vi "ScanFSM_v2.vi"(0 "Scan XY Map References":T3, 4 "Scan XY Map Handles":T2, 10 "Params XY Map SubVI":T7, 12 "Scan XY Map Exp Params SubVI":T6) -> (13 "Handles Out":T1, 16 "Data":i32[][](array[numeric]))   [LabVIEW 2019]
uses:
  TypeDefs/AcqMode.ctl
  Light Field/lightfield-automation-labview/LightField Automation.lvclass
panel:
  out "size(s)":i32[](array[numeric])
  out "Numeric 2":i32
  out "Numeric":i32
  out "Number of points":dbl=121.0
  out "YMultiplier":dbl
  out "YOffset":dbl
  out "XMultiplier":dbl
  out "XOffset":dbl
  out "XYPos Indices Randomized":dbl[][](array[numeric])
  out "XYPos Indices":i32[][](array[numeric])
  out "Random index":i32[](array[numeric])=[4, 16, 17, 14, 92, 29, 8, 31, 42, 104, 84, 28, 85, 90, 13, 60, 120, 41, 111, 82, 69, 34, 7, 77, 47, 59, 65, 116, 24, 30, 113, 2, 63, 94, 106, 103, 71, 100, 22, 18, 32, 102, 19, 97, 44, 12, 0, 1, 109, 27, 88, 99, 51, 107, 76, 56, 81, 96, 72, 93, 74, 21, 5, 79, 9, 117, 38, 45, 25, 58, 105, 57, 40, 52, 23, 87, 89, 62, 26, 110, 37, 3, 101, 10, 54, 61, 83, 46, 86, 66, 68, 43, 108, 11, 67, 75, 6, 80, 49, 20, 112, 78, 115, 119, 95, 64, 73, 39, 15, 48, 55, 70, 50, 98, 91, 35, 53, 36, 118, 33, 114]
  out "X size":dbl=11.0
  out "Y size":dbl=11.0
  out "WL Calib":dbl[](array[numeric])
  out "LF Error Out":errorcluster
  out "LF Out":refnum<class "LightField Automation.lvclass">
  out "CCD 1D Spectrum XY Map":refnum<vi>
  out "CCD 1D Spectrum XY Map 2":cluster{dbl[], dbl[]}(graph)
  out "CCD ROI":T4(ring)
  out "Accumulations":dbl
  out "Acq Mode":T5=enum."Spectrum"
  out "KCube Shutter On?":bool
  out "A Time (ms)":dbl
  out "XY Intensity Map":refnum<vi>
  out "XY Intensity Map":dbl[][](graph)=[[3.904687043201515e-13, 6.684989195773002e-11, 3.649880430807626e-09, 6.355065252727497e-08, 3.5287820878809013e-07, 6.248749509463085e-07, 3.5287820878809013e-07, 6.355065252727497e-08, 3.649880430807626e-09, 6.684989195773002e-11, 3.904687043201515e-13], [6.684989195773002e-11, 1.1444983952148092e-08, 6.248749509463097e-07, 1.0880140221963334e-05, 6.041424029819161e-05, 0.0001069812317752422, 6.041424029819161e-05, 1.0880140221963334e-05, 6.248749509463097e-07, 1.1444983952148092e-08, 6.684989195773002e-11], [3.649880430807626e-09, 6.248749509463097e-07, 3.41170163237202e-05, 0.0005940355282204004, 0.003298505755939091, 0.005840977343195246, 0.003298505755939091, 0.0005940355282204004, 3.41170163237202e-05, 6.248749509463097e-07, 3.649880430807626e-09], [6.355065252727497e-08, 1.0880140221963334e-05, 0.0005940355282204004, 0.01034317319661825, 0.05743261926761737, 0.10170139230422684, 0.05743261926761737, 0.01034317319661825, 0.0005940355282204004, 1.0880140221963334e-05, 6.355065252727497e-08], [3.5287820878809013e-07, 6.041424029819161e-05, 0.003298505755939091, 0.05743261926761737, 0.31890655732397044, 0.5647181220077593, 0.31890655732397044, 0.05743261926761737, 0.003298505755939091, 6.041424029819161e-05, 3.5287820878809013e-07], [6.248749509463085e-07, 0.0001069812317752422, 0.005840977343195246, 0.10170139230422684, 0.5647181220077593, 1.0, 0.5647181220077593, 0.10170139230422684, 0.005840977343195246, 0.0001069812317752422, 6.248749509463085e-07], [3.5287820878809013e-07, 6.041424029819161e-05, 0.003298505755939091, 0.05743261926761737, 0.31890655732397044, 0.5647181220077593, 0.31890655732397044, 0.05743261926761737, 0.003298505755939091, 6.041424029819161e-05, 3.5287820878809013e-07], [6.355065252727497e-08, 1.0880140221963334e-05, 0.0005940355282204004, 0.01034317319661825, 0.05743261926761737, 0.10170139230422684, 0.05743261926761737, 0.01034317319661825, 0.0005940355282204004, 1.0880140221963334e-05, 6.355065252727497e-08], [3.649880430807626e-09, 6.248749509463097e-07, 3.41170163237202e-05, 0.0005940355282204004, 0.003298505755939091, 0.005840977343195246, 0.003298505755939091, 0.0005940355282204004, 3.41170163237202e-05, 6.248749509463097e-07, 3.649880430807626e-09], [6.684989195773002e-11, 1.1444983952148092e-08, 6.248749509463097e-07, 1.0880140221963334e-05, 6.041424029819161e-05, 0.0001069812317752422, 6.041424029819161e-05, 1.0880140221963334e-05, 6.248749509463097e-07, 1.1444983952148092e-08, 6.684989195773002e-11], [3.904687043201515e-13, 6.684989195773002e-11, 3.649880430807626e-09, 6.355065252727497e-08, 3.5287820878809013e-07, 6.248749509463085e-07, 3.5287820878809013e-07, 6.355065252727497e-08, 3.649880430807626e-09, 6.684989195773002e-11, 3.904687043201515e-13]]
  out "XY Map Elapsed (s)":refnum<vi>
  out "XY Map Expected (s)":refnum<vi>
  out "XY Map Expected (s)":dbl caption="Expected (s)"
  out "XY Map Elapsed (s)":dbl caption="Elapsed (s)"
  in  "DigNum Refnum":refnum<vi>
  out "Scan XY Map Progess Bar":refnum<vi>
  out "Stop XY Map":refnum<vi>
  in  "CCD 2D Image XY Map":refnum<vi>
  out "Scan Y Readout (V)":refnum<vi>
  out "Scan X Readout (V)":refnum<vi>
  out "XYPositions":dbl[][](array[numeric])=[[-0.09999999999999998, -0.3], [-0.09999999999999998, -0.19999999999999996], [-0.3, 0.4], [0.20000000000000007, -0.09999999999999998], [-0.5, -0.5], [0.0, 0.20000000000000007], [0.30000000000000004, 0.30000000000000004], [-0.3, -0.5], [-0.5, 0.10000000000000009], [0.0, 0.4], [0.20000000000000007, 0.10000000000000009], [0.30000000000000004, 0.0], [-0.09999999999999998, -0.4], [-0.4, -0.19999999999999996], [-0.5, -0.19999999999999996], [0.4, 0.4], [-0.5, -0.4], [-0.5, -0.3], [-0.19999999999999996, 0.10000000000000009], [-0.19999999999999996, 0.4], [0.4, -0.5], [0.0, 0.10000000000000009], [-0.19999999999999996, 0.0], [0.10000000000000009, 0.30000000000000004], [-0.3, 0.10000000000000009], [0.10000000000000009, -0.3], [0.20000000000000007, -0.4], [-0.09999999999999998, 0.0], [-0.4, -0.5], [-0.5, 0.0], [-0.3, 0.20000000000000007], [-0.5, 0.20000000000000007], [-0.19999999999999996, 0.20000000000000007], [0.5, 0.4], [-0.4, 0.5], [0.5, 0.0], [0.5, 0.20000000000000007], [0.20000000000000007, -0.19999999999999996], [0.10000000000000009, -0.5], [0.4, 0.30000000000000004], [0.10000000000000009, 0.10000000000000009], [-0.4, 0.10000000000000009], [-0.5, 0.30000000000000004], [0.30000000000000004, -0.19999999999999996], [-0.09999999999999998, -0.5], [0.10000000000000009, -0.4], [0.20000000000000007, 0.5], [-0.3, -0.3], [0.4, 0.5], [0.30000000000000004, 0.5], [0.5, -0.3], [-0.09999999999999998, 0.30000000000000004], [0.10000000000000009, 0.20000000000000007], [0.5, 0.10000000000000009], [0.20000000000000007, 0.20000000000000007], [0.5, -0.5], [0.0, -0.5], [0.10000000000000009, 0.0], [0.10000000000000009, -0.19999999999999996], [-0.3, -0.19999999999999996], [-0.4, -0.09999999999999998], [0.20000000000000007, 0.30000000000000004], [0.20000000000000007, -0.5], [-0.3, 0.5], [0.4, 0.10000000000000009], [-0.3, -0.09999999999999998], [0.30000000000000004, -0.4], [0.30000000000000004, 0.10000000000000009], [0.30000000000000004, -0.3], [-0.4, 0.4], [0.5, -0.4], [-0.19999999999999996, -0.19999999999999996], [0.0, -0.19999999999999996], [0.4, 0.20000000000000007], [0.0, 0.0], [0.30000000000000004, 0.20000000000000007], [-0.09999999999999998, 0.5], [-0.3, -0.4], [0.4, -0.3], [0.0, 0.30000000000000004], [0.30000000000000004, 0.4], [0.0, -0.4], [-0.4, 0.30000000000000004], [0.20000000000000007, 0.4], [-0.5, 0.5], [-0.4, -0.4], [0.30000000000000004, -0.5], [0.10000000000000009, 0.4], [-0.09999999999999998, 0.10000000000000009], [0.10000000000000009, 0.5], [-0.4, -0.3], [0.5, -0.09999999999999998], [-0.5, -0.09999999999999998], [0.0, -0.09999999999999998], [-0.19999999999999996, -0.5], [0.4, 0.0], [0.0, -0.3], [-0.19999999999999996, 0.5], [0.5, -0.19999999999999996], [-0.09999999999999998, 0.20000000000000007], [-0.19999999999999996, -0.09999999999999998], [0.20000000000000007, 0.0], [-0.19999999999999996, 0.30000000000000004], [-0.19999999999999996, -0.3], [-0.5, 0.4], [0.10000000000000009, -0.09999999999999998], [-0.19999999999999996, -0.4], [-0.09999999999999998, 0.4], [0.30000000000000004, -0.09999999999999998], [-0.09999999999999998, -0.09999999999999998], [0.20000000000000007, -0.3], [-0.4, 0.20000000000000007], [0.4, -0.4], [-0.3, 0.30000000000000004], [0.5, 0.5], [0.4, -0.19999999999999996], [-0.3, 0.0], [0.0, 0.5], [0.5, 0.30000000000000004], [0.4, -0.09999999999999998], [-0.4, 0.0]]
  out "FSM X Task":refnum<k21>
  out "FSM Y Task":refnum<k21>
  out "Scan Y Res. (V)":dbl caption="Res. Y (V)"
  out "Scan Y Tot. Length":dbl caption="Y Length"
  out "Scan Y Center (V)":dbl caption="Y Center (V)"
  out "Scan Fast Axis":enum16{"Y", "X"}(ring)=enum."X" caption="Fast Axis"
  out "Scan X Res. (V)":dbl caption="Res. X (V)"
  out "Scan X Center (V)":dbl caption="X Center (V)"
  out "Scan X Tot. Length (V)":dbl caption="X Length (V)"
  out "Scanning Mode":T8(ring) caption="Mode"
  in  "Stop XY Map":bool
  out "Scan XY Map Progess Bar":u8(slide) scale=0.0..100.0
  out "CCD 2D Image XY Map":dbl[][](graph)
  out "Scan X Readout (V)":dbl caption="X Readout (V)" min=-10.0 max=10.0
  out "Scan Y Readout (V)":dbl caption="Y Readout (V)" min=-10.0 max=10.0
types:
  T1 = cluster{"LightField Automation out":refnum<class "LightField Automation.lvclass">, "error out":errorcluster, "FSM X Task":refnum<k21>, "FSM Y Task":refnum<k21>}
  T2 = cluster{"LightField Automation out":refnum<class "LightField Automation.lvclass">, "LightField Automation error out":errorcluster, "FSM X Task":refnum<k21>, "FSM Y Task":refnum<k21>}
  T3 = cluster{"Scan Main Progess Bar":refnum<vi>, "Acquire XY Map":refnum<vi>, "Pause XY Map":refnum<vi>, "Stop XY Map":refnum<vi>, "Save XY Map":refnum<vi>, "Scan X Readout (V)":refnum<vi>, "Scan Y Readout (V)":refnum<vi>, "CCD 1D Spectrum XY Map":refnum<vi>, "XY Intensity Map":refnum<vi>, "CCD 2D Image XY Map":refnum<vi>, "XY Map Expected (s)":refnum<vi>, "XY Map Elapsed (s)":refnum<vi>}
  T4 = enum16{"Custom ROI", "Full sensor", "Binned full sensor"}
  T5 = typedef "AcqMode.ctl" = enum16{"Image", "Spectrum", "APD 1", "APD 2", "APD 1+2"}
  T6 = cluster{"Exposure Time (ms)":dbl, "Accumulations":dbl, "Excitation Wavelength (nm)":dbl, "Acq Mode":T5, "CCD ROI":enum16{"Custom ROI", "Full sensor", "Binned full sensor"}, "KCube Shutter On?":bool}
  T7 = cluster{"Scan Fast Axis":enum16{"Y", "X"}, "Scanning Mode":enum16{"Default", "Snail", "Random", "Snake", "Line"}, "Scan X Center (V)":dbl, "Scan X Res. (V)":dbl, "Scan X Tot. Length (V)":dbl, "Scan Y Center (V)":dbl, "Scan Y Res. (V)":dbl, "Scan Y Tot. Length":dbl}
  T8 = enum16{"Default", "Snail", "Random", "Snake", "Line"}
  T9 = enum16{"Image", "Spectrum", "APD 1", "APD 2", "APD 1+2"}
  T10 = enum16{"Contrast", "Spectre", "Polarisation", "Time Trace", "XY Intensity Map"}
  T11 = cluster{"Image":dbl[][][], "Frame Size":cluster{"F":i32, "Y":i32, "X":i32}}[]
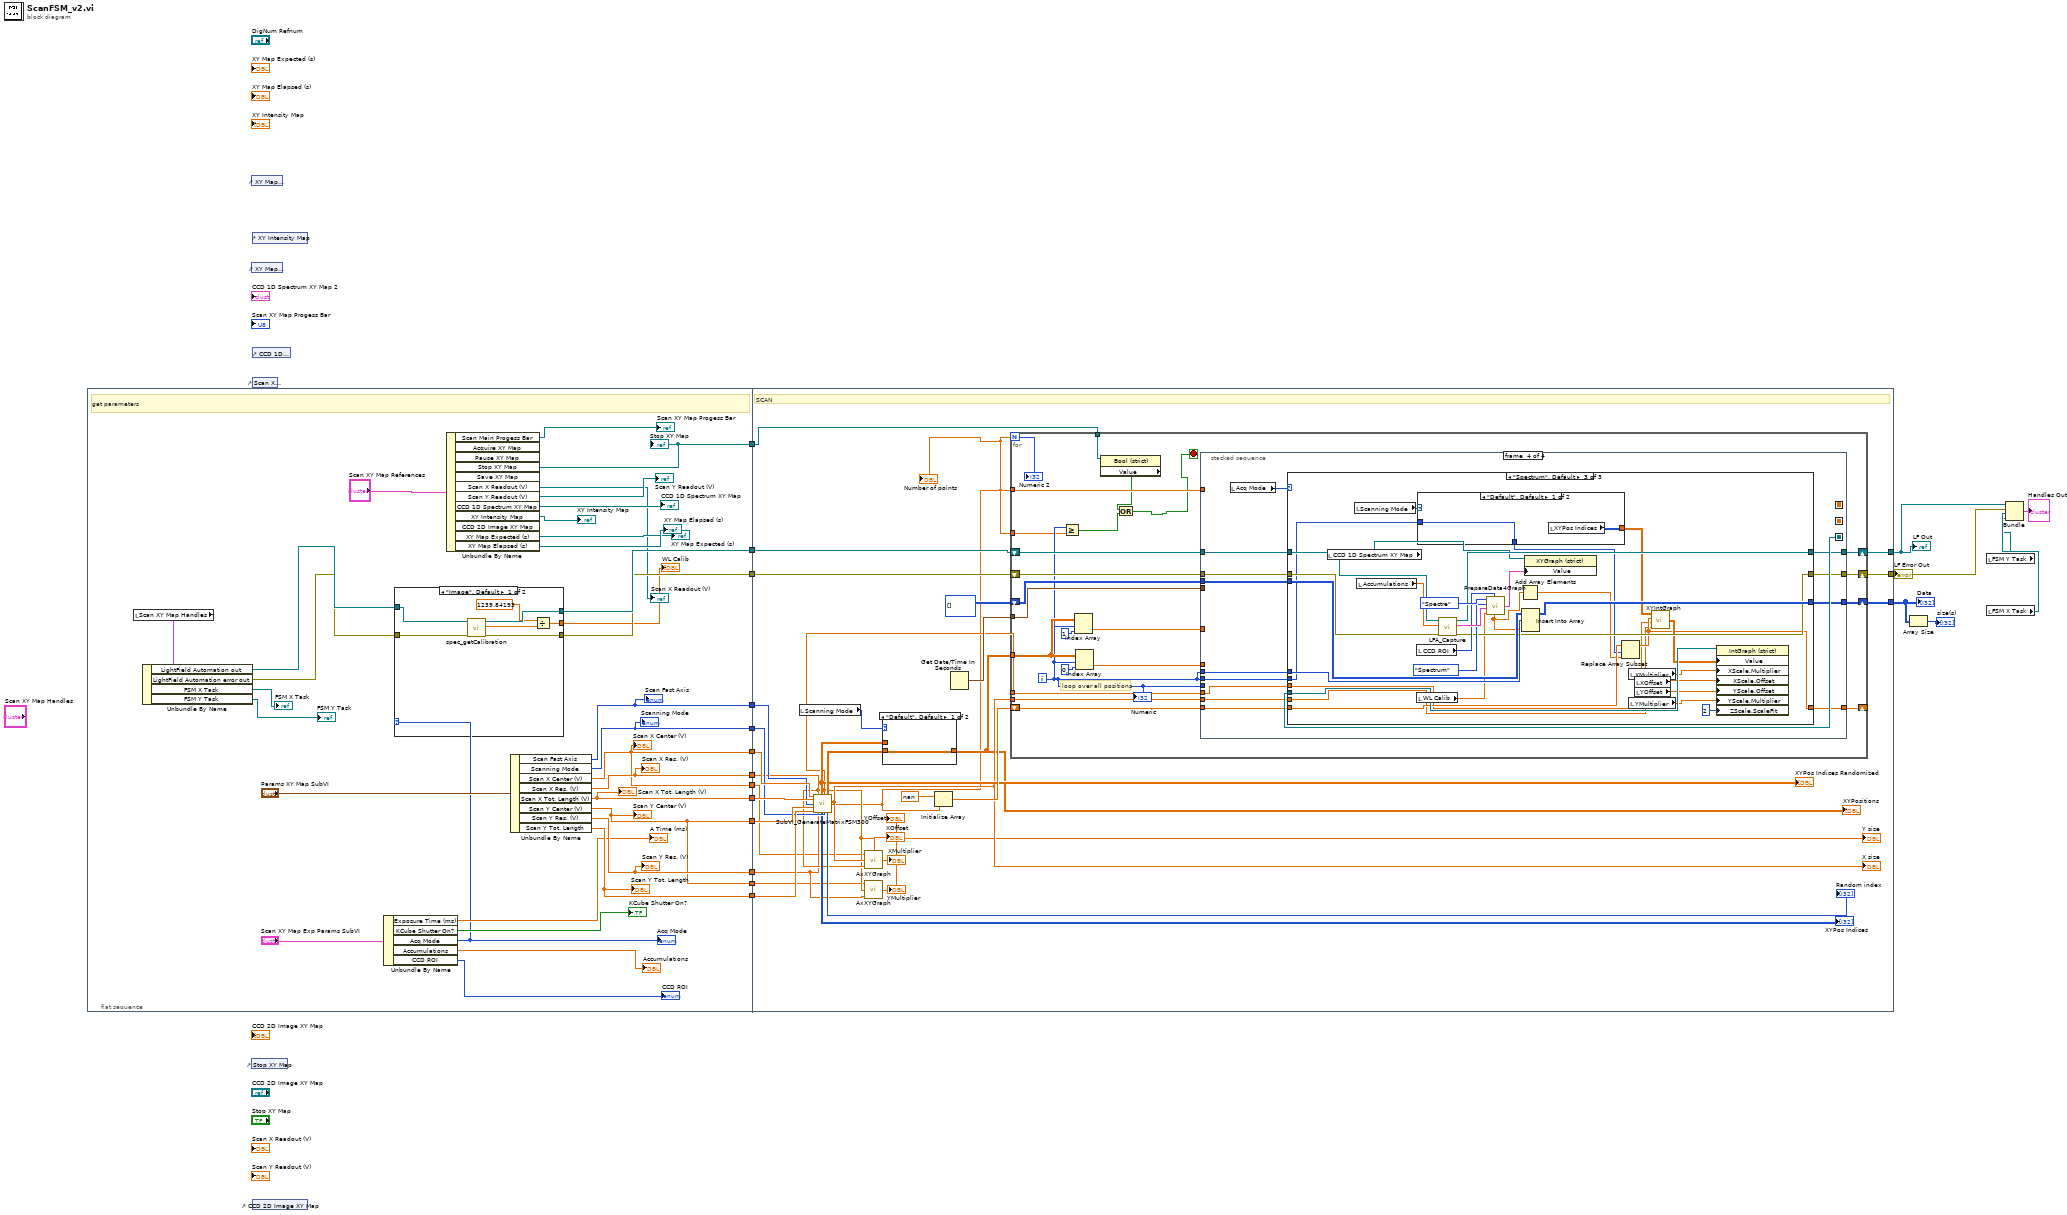
[diagram p0: block diagram]
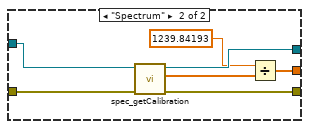
[diagram p2: hidden frame]
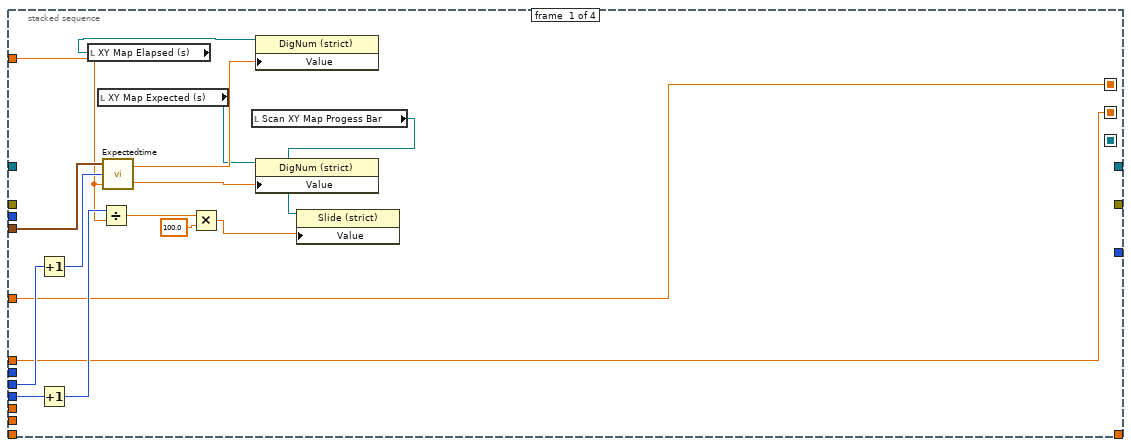
[diagram p4: hidden frame]
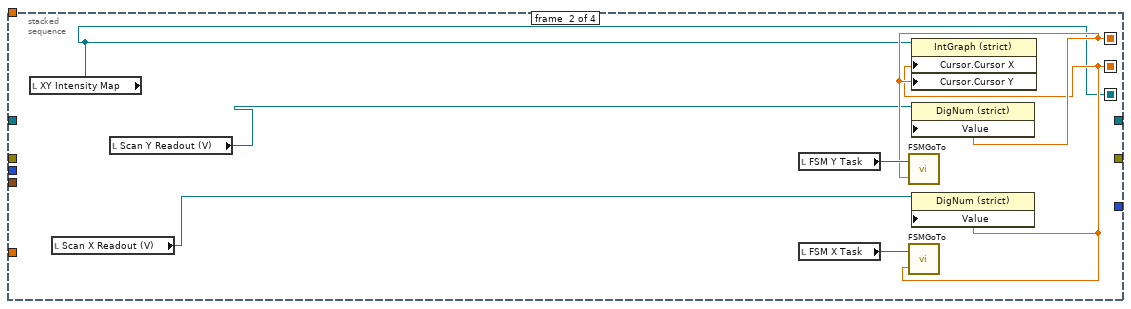
[diagram p5: hidden frame]
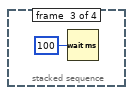
[diagram p6: hidden frame]
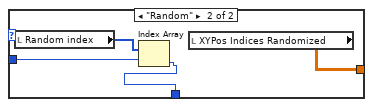
[diagram p9: hidden frame]
diagram:
  n1 = flat-sequence {
    tunnel: [w51] -> w20
    tunnel: [w36] -> w19
    tunnel: [w50] -> w18
    tunnel: [w49] -> w17
    tunnel: [w35] -> w16
    tunnel: [w48] -> w15
    tunnel: [w47] -> w14
    tunnel: [w46] -> w13
    tunnel: [w39] -> w12
    tunnel: [w38] -> w11
    tunnel: [w36] -> w10
    tunnel: [w35] -> w9
    tunnel: [w33] -> w6
    tunnel: w20 -> [w79]
    tunnel: w19 -> [w98]
    tunnel: w18 -> [w97]
    tunnel: w17 -> [w96]
    tunnel: w16 -> [w95]
    tunnel: w15 -> [w94]
    tunnel: w14 -> [w75]
    tunnel: w13 -> [w93]
    tunnel: [w91] -> w8
    tunnel: [w90] -> w5
    tunnel: [w89] -> w4
    tunnel: w12 -> [w88]
    tunnel: w11 -> [w87]
    tunnel: w10 -> [w72]
    tunnel: w9 -> [w71]
    tunnel: w6 -> [w67]
    frame #0 {
      # "get parameters"
      n2 = local read "Scan XY Map Handles"() -> (w25:T2)
      n3 = Unbundle By Name(w25) -> ("LightField Automation out"=w24:refnum<class "LightField Automation.lvclass">, "LightField Automation error out"=w23:errorcluster, "FSM X Task"=→"FSM X Task":refnum<k21>, "FSM Y Task"=→"FSM Y Task":refnum<k21>)
      n4 = Unbundle By Name("Scan XY Map Exp Params SubVI") -> ("Exposure Time (ms)"=→"A Time (ms)":dbl, "KCube Shutter On?"=→"KCube Shutter On?":bool, "Acq Mode"=w40:T5, "Accumulations"=→"Accumulations":dbl, "CCD ROI"=→"CCD ROI":T4)
      "Acq Mode" <- w40
      n5 = case shown="\"Image\", Default" w40 {
        tunnel: w24 -> [w59 w66]
        tunnel: w23 -> [w58 w65]
        tunnel: [w57 w64] -> w39
        tunnel: [w56 w63] -> w38
        tunnel: [w53 w60] -> w37
        frame "Image", Default {
          n6 = call "spec_getCalibration.vi"("error in (no error)"=w58, "LightField Automation in"=w59) -> ("error out"=w56:errorcluster, "ColumnCalibration"=w54:dbl[], "LightField Automation out"=w57:refnum<class "LightField Automation.lvclass">)  [unwired: 7 in]
          n7 = Divide(x=1239.84193, y=w54) -> (x/y=w53:dbl[])
        }
        frame "Spectrum" {
          n8 = call "spec_getCalibration.vi"("error in (no error)"=w65, "LightField Automation in"=w66) -> ("error out"=w63:errorcluster, "ColumnCalibration"=w61:dbl[], "LightField Automation out"=w64:refnum<class "LightField Automation.lvclass">)  [unwired: 7 in]
          n9 = Divide(x=1239.84193, y=w61) -> (x/y=w60:dbl[])
        }
      }
      "WL Calib" <- w37
      n10 = Unbundle By Name("Scan XY Map References") -> ("Scan Main Progess Bar"=→"Scan XY Map Progess Bar":refnum<vi>, "Stop XY Map"=w33:refnum<vi>, "Scan X Readout (V)"=→"Scan X Readout (V)":refnum<vi>, "Scan Y Readout (V)"=→"Scan Y Readout (V)":refnum<vi>, "CCD 1D Spectrum XY Map"=→"CCD 1D Spectrum XY Map":refnum<vi>, "XY Intensity Map"=→"XY Intensity Map":refnum<vi>, "XY Map Expected (s)"=→"XY Map Expected (s)":refnum<vi>, "XY Map Elapsed (s)"=→"XY Map Elapsed (s)":refnum<vi>)  [unwired: 4 out]
      "Stop XY Map" <- w33
      n11 = Unbundle By Name("Params XY Map SubVI") -> ("Scan Fast Axis"=w49:enum16{"Y", "X"}, "Scanning Mode"=w46:T8, "Scan X Center (V)"=w36:dbl, "Scan X Res. (V)"=w51:dbl, "Scan X Tot. Length (V)"=w50:dbl, "Scan Y Center (V)"=w35:dbl, "Scan Y Res. (V)"=w47:dbl, "Scan Y Tot. Length"=w48:dbl)
      "Scan X Tot. Length (V)" <- w50
      "Scan X Res. (V)" <- w51
      "Scan Y Center (V)" <- w35
      "Scan Y Tot. Length" <- w48
      "Scan Y Res. (V)" <- w47
      "Scanning Mode" <- w46
      "Scan X Center (V)" <- w36
      "Scan Fast Axis" <- w49
    }
    frame #1 {
      # "SCAN"
      n12 = local read "Scanning Mode"() -> (w83:T8)
      n13 = call "SubVI_GenerateMatrixFSM300.vi"("X center (Volt)"=w98, "Total Length X (Volt)"=w97, "''fast mooving'' axis"=w96, "Y center (Volt)"=w95, "Total Length Y (Volt)"=w94, "Resolution X (Volt)"=w79, "Resolution Y (Volt)"=w75, "Scan mode"=w93) -> ("XYPos Indices Randomized"=w81:dbl[][], "XYPos Indices"=→"XYPos Indices":i32[][], "Y size"=w76:dbl, "XYPositions"=w82:dbl[][], "Random index"=→"Random index":i32[], "X size"=w80:dbl, "Number of points"=w69:dbl)  [unwired: 1 in, 4 out]
      "Y size" <- w76
      "X size" <- w80
      "XYPos Indices Randomized" <- w81
      "Number of points" <- w69
      n14 = call "AxXYGraph.vi"("dx"=w79, "N"=w80, "x0"=w72) -> ("Multiplier"=→"XMultiplier":dbl, "Offset"=→"XOffset":dbl)
      n15 = call "AxXYGraph.vi"("dx"=w75, "N"=w76, "x0"=w71) -> ("Multiplier"=→"YMultiplier":dbl, "Offset"=→"YOffset":dbl)
      n16 = case shown="\"Default\", Default" w83 {
        tunnel: w82 -> [w100 w101]
        tunnel: [w100 w101] -> w70
        tunnel: w81 -> [_ _]
        frame "Default", Default {
        }
        frame "Random" {
        }
      }
      "XYPositions" <- w70
      n17 = Initialize Array(nan, w69) -> (w85:dbl[])
      n18 = Get Date/Time In Seconds() -> (seconds since 1Jan1904=w99:timestamp)
      n19 = for {
        N: w69 -> [w108]
        tunnel: w70 -> [w125]
        tunnel: w99 -> [w120]
        shift-right: [w118] -> w91
        shift-left: i32[][] [] -> [w119]
        shift-right: [w117] -> w90
        shift-left: w88 -> [w116]
        shift-right: [w114] -> w89
        shift-left: w87 -> [w115]
        shift-right: [w112] -> _
        shift-left: w85 -> [w113]
        tunnel: w80 -> [w111]
        tunnel: w76 -> [w110]
        tunnel: w69 -> [w109]
        tunnel: w69 -> [w106]
        tunnel: w67 -> [w102]
        i -> [w107]
        stop <- w103 stop-if-true
        # "loop over all positions"
        n20 = Greater Or Equal?(x=w107, y=w106) -> (x >= y?=w105:bool)
        n21 = Index Array(array=w125, index (row)=w107, index (col)=1 ("index")) -> (element=w122:dbl)
        n22 = Index Array(array=w125, index (row)=w107, index (col)=0 ("index")) -> (element=w121:dbl)
        n23 = property class="Bool (strict)"(reference=w102) -> ("Value"=w104:bool)  [unwired: 1 in, 2 out]
        n24 = Or(x=w104, y=w105) -> (x .or. y?=w103:bool)
        n25 = stacked-sequence {
          seq-local: [w131 _ _ _] -> [_ w146 _ _]
          seq-local: [w130 _ _ _] -> [_ w145 _ _]
          seq-local: [_ w142 _ _] -> [_ _ _ w162]
          tunnel: w122 -> [w131 _ _ _]
          tunnel: w121 -> [w130 _ _ _]
          tunnel: w107 -> [w141 _ _ _]
          tunnel: w109 -> [w134 _ _ _]
          tunnel: w120 -> [w137 _ _ _]
          tunnel: w107 -> [w136 _ _ w153]
          tunnel: w119 -> [_ _ _ w161]
          tunnel: w107 -> [_ _ _ w160]
          tunnel: [_ _ _ w159] -> w118
          tunnel: [_ _ _ w158] -> w117
          tunnel: w116 -> [_ _ _ w157]
          tunnel: w115 -> [_ _ _ w156]
          tunnel: [_ _ _ w155] -> w114
          tunnel: w113 -> [_ _ _ w154]
          tunnel: [_ _ _ w152] -> w112
          tunnel: w111 -> [_ _ _ w151]
          tunnel: w110 -> [_ _ _ w150]
          frame #0 {
            n26 = Increment(x=w136) -> (x+1=w135:i32)
            n27 = Increment(x=w141) -> (x+1=w140:i32)
            n28 = local read "XY Map Elapsed (s)"() -> (w128:refnum<vi>)
            n29 = local read "XY Map Expected (s)"() -> (w127:refnum<vi>)
            n30 = Divide(x=w140, y=w134) -> (x/y=w139:dbl)
            n31 = call "Expectedtime.vi"("N"=w134, "I"=w135, "Reference time"=w137) -> ("Expected time"=w133:dbl, "Elapsed time"=w132:dbl)
            n32 = Multiply(x=w139, y=100.0 ("x/y")) -> (x*y=w129:dbl)
            n33 = local read "Scan XY Map Progess Bar"() -> (w126:refnum<vi>)
            n34 = property class="DigNum (strict)"(reference=w128, "Value"=w132) -> ()  [unwired: 1 in, 2 out]
            n35 = property class="DigNum (strict)"(reference=w127, "Value"=w133) -> ()  [unwired: 1 in, 2 out]
            n36 = property class="Slide (strict)"(reference=w126, "Value"=w129) -> ()  [unwired: 1 in, 2 out]
          }
          frame #1 {
            n37 = local read "XY Intensity Map"() -> (w142:refnum<vi>)
            n38 = local read "Scan X Readout (V)"() -> (w143:refnum<vi>)
            n39 = local read "Scan Y Readout (V)"() -> (w144:refnum<vi>)
            n40 = local read "FSM Y Task"() -> (w148:refnum<k21>)
            n41 = local read "FSM X Task"() -> (w147:refnum<k21>)
            n42 = call "FSMGoTo.vi"("Target Value (V)"=w146, "FSM Task"=w148) -> ()  [unwired: 1 out]
            n43 = call "FSMGoTo.vi"("Target Value (V)"=w145, "FSM Task"=w147) -> ()  [unwired: 1 out]
            n44 = property class="IntGraph (strict)"(reference=w142, "Cursor.Cursor X"=w145, "Cursor.Cursor Y"=w146) -> ()  [unwired: 1 in, 2 out]
            n45 = property class="DigNum (strict)"(reference=w144, "Value"=w146) -> ()  [unwired: 1 in, 2 out]
            n46 = property class="DigNum (strict)"(reference=w143, "Value"=w145) -> ()  [unwired: 1 in, 2 out]
          }
          frame #2 {
            n47 = Wait (ms)(milliseconds to wait=u32 100) -> ()  [unwired: 1 out]
          }
          frame #3 {
            n48 = local read "Acq Mode"() -> (w163:T5)
            n49 = case shown="\"Spectrum\", Default" w163 {
              tunnel: w157 -> [w166 w170 w203]
              tunnel: w156 -> [w165 w169 w202]
              tunnel: w162 -> [_ _ w196]
              tunnel: w161 -> [w167 w171 w194]
              tunnel: w160 -> [_ _ w193]
              tunnel: [w167 w171 w192] -> w159
              tunnel: [w166 w170 w191] -> w158
              tunnel: [w165 w169 w190] -> w155
              tunnel: w154 -> [w164 w168 w187]
              tunnel: w153 -> [_ _ w175]
              tunnel: [w164 w168 w184] -> w152
              tunnel: w151 -> [_ _ w176]
              tunnel: w150 -> [_ _ w183]
              frame "Image" {
              }
              frame "APD 1" {
              }
              frame "Spectrum", Default {
                n50 = local read "CCD 1D Spectrum XY Map"() -> (w172:refnum<vi>)
                n51 = local read "Scanning Mode"() -> (w182:T8)
                n52 = local read "Accumulations"() -> (w201:dbl)
                n53 = local read "CCD ROI"() -> (w197:T4)
                n54 = local read "WL Calib"() -> (w189:dbl[])
                n55 = case shown="\"Default\", Default" w182 {
                  tunnel: [w205 w209] -> w181
                  tunnel: w175 -> [w204 w207]
                  tunnel: [w204 w206] -> w174
                  frame "Default", Default {
                    n56 = local read "XYPos Indices"() -> (w205:i32[][])
                  }
                  frame "Random" {
                    n57 = local read "Random index"() -> (w208:i32[])
                    n58 = Index Array(array=w208, index=w207) -> (element=w206:i32)
                    n59 = local read "XYPos Indices Randomized"() -> (w209:dbl[][])
                  }
                }
                n60 = call "LFA_Capture.vi"("error in (no error)"=w202, "Frames"=w201, "LightField Automation in"=w203) -> ("error out"=w190:errorcluster, "Data"=w200:T11, "LightField Automation out"=w191:refnum<class "LightField Automation.lvclass">)  [unwired: 6 in]
                n61 = call "PrepareData4Graph.vi"("Wavelength nm"=w189, "DataLF"=w200, "CCD ROI"=w197, "AcqMode"=T9."Spectrum", "Data type"=T10."Spectre") -> ("Spectrum"=w195:cluster{"Array 2":dbl[], "Array":dbl[]}, "PLInt out"=w186:dbl[])  [unwired: 2 in, 2 out]
                n62 = Add Array Elements(numeric array=w186) -> (sum=w185:dbl)
                n63 = Insert Into Array(array=w194, index (row)=w193, new element=w186) -> (w192:i32[][])  [unwired: 1 in]
                n64 = property class="XYGraph (strict)"(reference=w172, "Value"=w195) -> ()  [unwired: 1 in, 2 out]
                n65 = Replace Array Subset(array=w187, new element=w185, index=w174) -> (w184:dbl[])
                n66 = local read "XMultiplier"() -> (w180:dbl)
                n67 = local read "YMultiplier"() -> (w177:dbl)
                n68 = local read "XOffset"() -> (w179:dbl)
                n69 = local read "YOffset"() -> (w178:dbl)
                n70 = call "XYIntGraph.vi"("Columns"=w176, "Rows"=w183, "Z Intensity"=w184, "XY Pos"=w181) -> ("Intensity Graph"=w188:dbl[][])
                n71 = property class="IntGraph (strict)"(reference=w196, "Value"=w188, "XScale.Multiplier"=w180, "XScale.Offset"=w179, "YScale.Offset"=w178, "YScale.Multiplier"=w177, "ZScale.ScaleFit"=u8 2 ("Z Scale.Scale Fit")) -> ()  [unwired: 1 in, 2 out]
              }
            }
          }
        }
        "Numeric" <- w107
        "Numeric 2" <- w108
      }
    }
  }
  n72 = control-ref of="XY Map Expected (s)"() -> ()  [unwired: 1 out]
  n73 = control-ref of="XY Map Elapsed (s)"() -> ()  [unwired: 1 out]
  n74 = control-ref of="Stop XY Map"() -> ()  [unwired: 1 out]
  n75 = control-ref of="Scan XY Map Progess Bar"() -> ()  [unwired: 1 out]
  n76 = control-ref of="XY Intensity Map"() -> ()  [unwired: 1 out]
  n77 = control-ref of="CCD 1D Spectrum XY Map"() -> ()  [unwired: 1 out]
  n78 = control-ref of="CCD 2D Image XY Map"() -> ()  [unwired: 1 out]
  n79 = Array Size(array=w8) -> (size(s)=→"size(s)":i32[])
  n80 = local read "FSM Y Task"() -> (w2:refnum<k21>)
  n81 = local read "FSM X Task"() -> (w3:refnum<k21>)
  n82 = Bundle("LightField Automation out"=w5, "error out"=w4, "FSM X Task"=w3, "FSM Y Task"=w2) -> (→"Handles Out":T1)  [unwired: 1 in]
  "Data" <- w8
  "LF Out" <- w5
  "LF Error Out" <- w4
